vi "Untitled 1.vi"() -> ()   [LabVIEW 2016]
uses:
  <vilib>/Platform/TimedLoop/XDataNode/timing_clust.ctl
  <vilib>/Platform/TimedLoop/XDataNode/nitl_modes.ctl
  <vilib>/Platform/TimedLoop/XDataNode/wakeup.ctl
  <vilib>/rvi/Emulation/niFpgaGetClockAttributes.vi
  <vilib>/rvi/Emulation/niFpgaSctlEmulationGetInTimedLoop.vi
  <vilib>/rvi/Emulation/niFpgaEmulationReportErrorSimple.vi
  <vilib>/rvi/Emulation/niFpgaCriticalErrorInLSC.vi
  <vilib>/rvi/eio/common/nirviEmuTemplateMethod_errors.vi
  <vilib>/platform/TimedLoop/XDataNode/XDataNode.xnode
  <vilib>/eio/EIONode/EIONode.xnode
  <vilib>/Platform/TimedLoop/XDataNode/XDNodeRunTimeDep.lvlib
panel:
  in  "Delay (Ticks)":u16 caption="Delay(Ticks)"
  in  "no triggers":u16=10
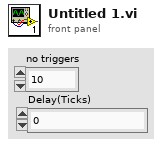
[diagram p1: front panel]
types:
  T1 = typedef "XDNodeRunTimeDep.lvlib/timing_clust.ctl" = cluster{"Expected End [f-1]":u64, "Actual End [f-1]":u64, "Finished Late? [f-1]":bool, "Expected End [i-1]":u64, "Actual End [i-1]":u64, "Finished Late? [i-1]":bool, "Expected Start [i]":u64, "Actual Start [i]":u64, "Expected Start [f]":u64, "Actual Start [f]":u64, "Source Name":string, "Structure Name":string, "Period":i64, "Deadline":i64, "Offset":i64, "Start":i64, "Priority":i32, "Timeout":i32, "Mode":T2, "Wakeup Reason":T3, "Error":errorcluster, "Source Type":string, "Secondary Source Type":string, "Global End Time":u64, "Global Start Time":u64, "Frame Duration":u64, "Iteration Duration":u64, "Assigned CPU":i32, "I/O Scan Engine Mode":u32}
  T2 = typedef "XDNodeRunTimeDep.lvlib/nitl_modes.ctl" = enum32{"No Change", "Process missed periods, maintain original phase", "Discard missed periods, maintain original phase", "Process missed periods, ignore original phase", "Discard missed periods, ignore original phase"}
  T3 = typedef "XDNodeRunTimeDep.lvlib/wakeup.ctl" = enum32{"Normal", "Aborted", "Asynchronous wakeup", "Timing source error", "Timed loop error", "Timeout"}
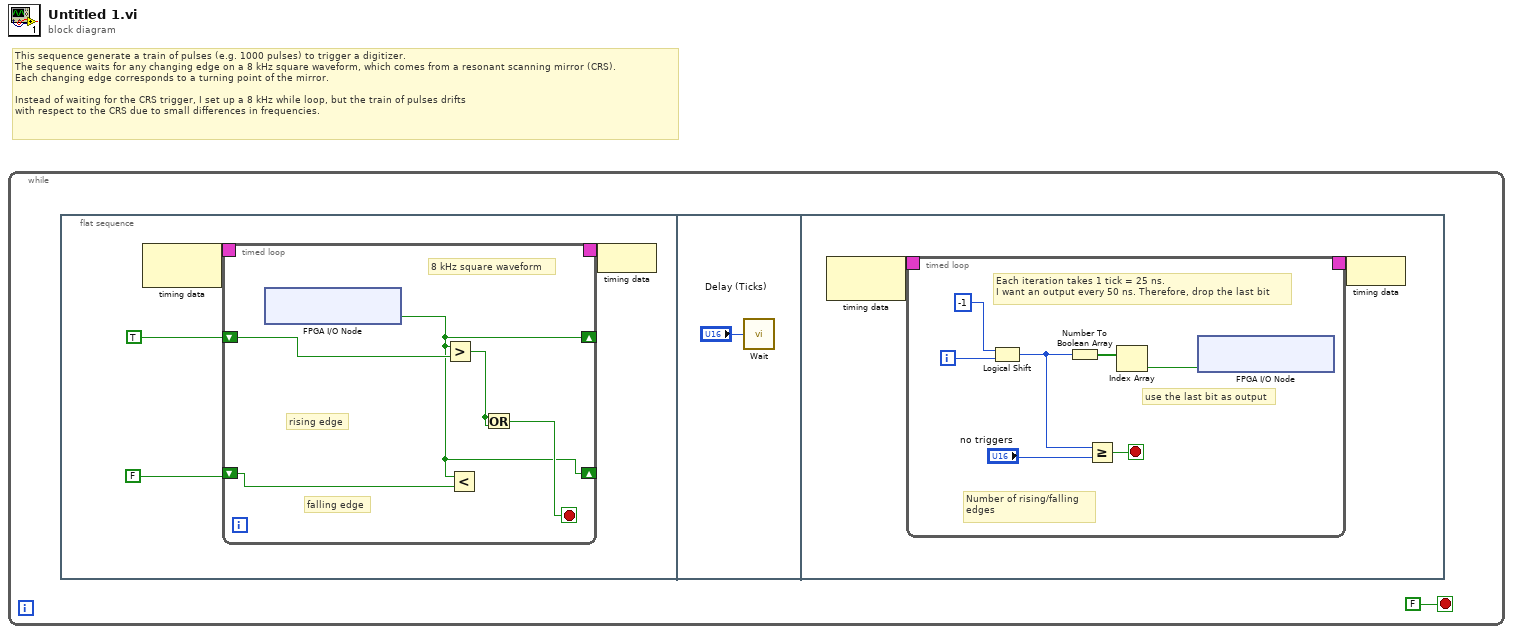
[diagram p0: block diagram]
diagram:
  # "This sequence generate a train of pulses (e.g. 1000 pulses) to trigger a digitizer.\nThe sequence waits for any changing edge on a 8 kHz square waveform, which comes from a resonant scanning mirror (CRS).\nEach changing edge corresponds to a turning point of the mirror.\n\nInstead of waiting for the CRS trigger, I set up a 8 kHz while loop, but the train of pulses drifts\nwith respect to the CRS due to small differences in frequencies."
  n1 = while {
    stop <- FALSE stop-if-true
    n2 = flat-sequence {
      frame #0 {
        n3 = node-c288() -> (w5:T1)  [unwired: 1 in]
        n4 = timed-loop {
          timing: w5 -> [_]
          timing-out: [_] -> w4
          shift-right: [w7] -> _
          shift-left: TRUE -> [w10]
          shift-right: [w7] -> _
          shift-left: FALSE -> [w8]
          stop <- w9 stop-if-true
          # "8 kHz square waveform"
          # "falling edge"
          # "rising edge"
          n5 = xnode "FPGA I/O Node"() -> ("Connector0/DIO0"=w7:bool)  [unwired: 1 in, 1 out]
          n6 = Greater?(x=w7, y=w10) -> (0:w6:bool)
          n7 = Less?(x=w7, y=w8) -> ()  [unwired: 1 out]
          n8 = Or(x=w6, y=w6) -> (x .or. y?=w9:bool)
        }
        n9 = node-c288(w4) -> ()
      }
      frame #1 {
        n10 = call "Wait"("Count(Ticks)"="Delay (Ticks)") -> ()  [unwired: 1 out]
      }
      frame #2 {
        n11 = node-c288() -> (w17:T1)  [unwired: 1 in]
        n12 = timed-loop {
          timing: w17 -> [_]
          timing-out: [_] -> w16
          i -> [w22]
          stop <- w24 stop-if-true
          # "Number of rising/falling\nedges"
          # "use the last bit as output"
          # "Each iteration takes 1 tick = 25 ns.\nI want an output every 50 ns. Therefore, drop the last bit"
          n13 = Logical Shift(y=i16 -1, x=w22) -> (x << y=w18:i32)
          n14 = Number To Boolean Array(number=w18) -> (Boolean array=w23:bool[])
          n15 = Greater Or Equal?(x=w18, y="no triggers") -> (x >= y?=w24:bool)
          n16 = Index Array(array=w23) -> (element=w19:bool)  [unwired: 1 in]
          n17 = xnode "FPGA I/O Node"("Connector0/DIO1"=w19) -> ()  [unwired: 1 in, 1 out]
        }
        n18 = node-c288(w16) -> ()
      }
    }
  }
